vi "PWM Split Control Lines (Single Output).vi"(11 "Counter Control":u8 format="%08b") -> (2 "Compare Output Mode":fxp<+,2,2> format="%02b", 3 "Waveform Generation Mode":fxp<+,2,2> format="%02b")   [LabVIEW 2014]
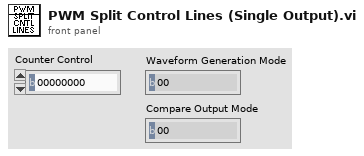
[diagram p1: front panel]
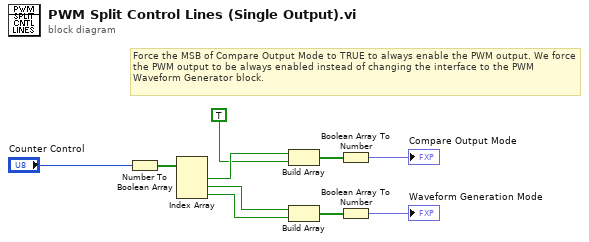
[diagram p0: block diagram]
diagram:
  # "Force the MSB of Compare Output Mode to TRUE to always enable the PWM output. We force the PWM output to be always enabled instead of changing the interface to the PWM Waveform Generator block."
  n1 = Number To Boolean Array(number="Counter Control") -> (Boolean array=w10:bool[])
  n2 = Index Array(array=w10) -> (element #1=w8:bool, element #2=w2:bool, element #3=w1:bool)  [unwired: 3 in]
  n3 = Build Array(w8, TRUE ("element")) -> (w7:bool[])
  n4 = Build Array(w2, w1) -> (w6:bool[])
  n5 = Boolean Array To Number(Boolean array=w7) -> (number=→"Compare Output Mode":fxp<+,2,2>)
  n6 = Boolean Array To Number(Boolean array=w6) -> (number=→"Waveform Generation Mode":fxp<+,2,2>)
